vi "Set Refs.vi"(8 "error in (no error)":errorcluster, 10 "Refs":T1, 11 "ExcuseNotes in":refnum<class "ExcuseNotesHandler.lvclass">) -> (0 "error out":errorcluster, 3 "ExcuseNotes out":refnum<class "ExcuseNotesHandler.lvclass">)   [LabVIEW 2015, in "Admin_Actor.lvlib" / "ExcuseNotesHandler.lvclass"]
uses:
  ExcuseNotesHandler.lvclass
  Type Definitions/Main Ctls And VI Refs.ctl
  ExcuseNotesHandler.lvclass/ExcuseNotesHandler.ctl
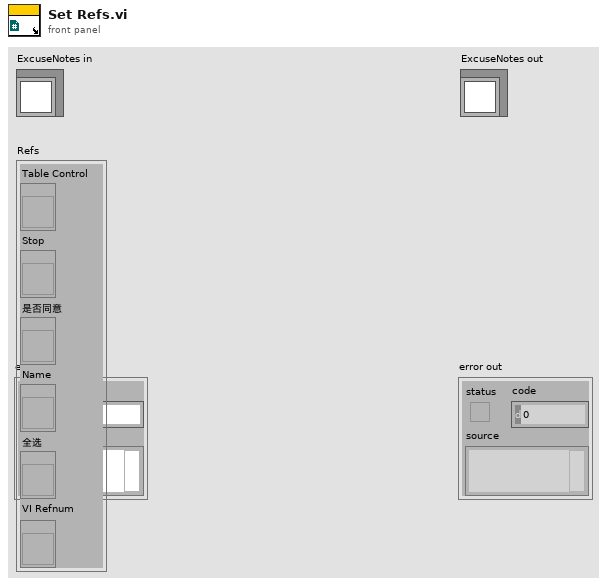
[diagram p1: front panel]
types:
  T1 = typedef "Admin_Actor.lvlib/ExcuseNotesHandler.lvclass/Main Ctls And VI Refs.ctl" = cluster{"Table Control":refnum<vi>, "Stop":refnum<vi>, "是否同意":refnum<vi>, "Name":refnum<vi>, "全选":refnum<vi>, "VI Refnum":refnum<vi>}
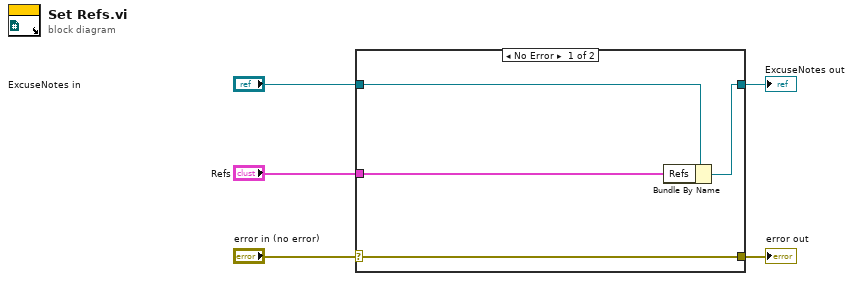
[diagram p0: block diagram]
diagram:
  n1 = case shown="No Error" "error in (no error)" {
    selector: "error in (no error)" -> [w9 w10]
    tunnel: [w9 w10] -> w4
    tunnel: [w7 w11] -> w2
    tunnel: "ExcuseNotes in" -> [w8 w11]
    tunnel: "Refs" -> [w6 _]
    frame No Error {
      n2 = Bundle By Name(cluster=w8, "Refs"=w6) -> (w7:refnum<class "ExcuseNotesHandler.lvclass">)
    }
    frame Error {
    }
  }
  "error out" <- w4
  "ExcuseNotes out" <- w2
